vi "Calculate Acceptance Probability.vi"(8 "error in (no error)":errorcluster, 11 "SA in":refnum<class "SA.lvclass">) -> (0 "error out":errorcluster, 2 "Acceptance Probability":dbl, 3 "SA out":refnum<class "SA.lvclass">)   [LabVIEW 2013, in "SA.lvclass"]
uses:
  SA.lvclass
  SA.lvclass/SA.ctl
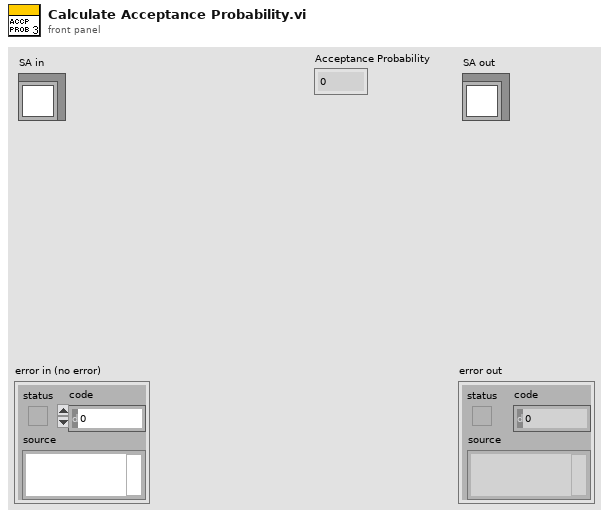
[diagram p1: front panel]
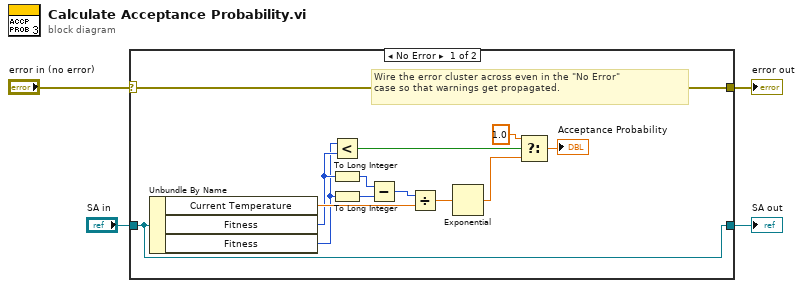
[diagram p0: block diagram]
diagram:
  n1 = case shown="No Error" "error in (no error)" {
    selector: "error in (no error)" -> [w17 w19]
    tunnel: [w17 w19] -> w3
    tunnel: [w16 w18] -> w1
    tunnel: "SA in" -> [w16 w18]
    frame No Error {
      # "Wire the error cluster across even in the \"No Error\"\ncase so that warnings get propagated."
      n2 = Unbundle By Name(w16) -> ("Current Temperature"=w12:dbl, "Fitness"=w8:u16, "Fitness"=w6:u16)
      n3 = Less?(x=w6, y=w8) -> (x < y?=w15:bool)
      n4 = To Long Integer(number=w8) -> (32bit integer=w7:i32)
      n5 = To Long Integer(number=w6) -> (32bit integer=w5:i32)
      n6 = Subtract(x=w7, y=w5) -> (x-y=w13:i32)
      n7 = Divide(x=w13, y=w12) -> (x/y=w11:dbl)
      n8 = Exponential(1:w11) -> (0:w10:dbl)
      n9 = Select(t=1.0, s=w15, f=w10) -> (s? t:f=→"Acceptance Probability":dbl)
    }
    frame Error {
    }
  }
  "error out" <- w3
  "SA out" <- w1
